vi "check_drift_during_experiment.vi"(8 "error in (no error)":errorcluster, 10 "Processed Image":T1(plugin-control), 11 "max spatial drift since calibration (mm)":dbl) -> (0 "error out":errorcluster, 1 "max spatial drift since experiment start (mm)":sgl, 2 "Image Out":T1, 3 "Warning needed":bool)   [LabVIEW 2019]
uses:
  <vilib>/vision/Image Controls.llb/IMAQ Image.ctl
  ParametersGlobal.vi
  <vilib>/vision/NI_Vision_Development_Module.lvlib
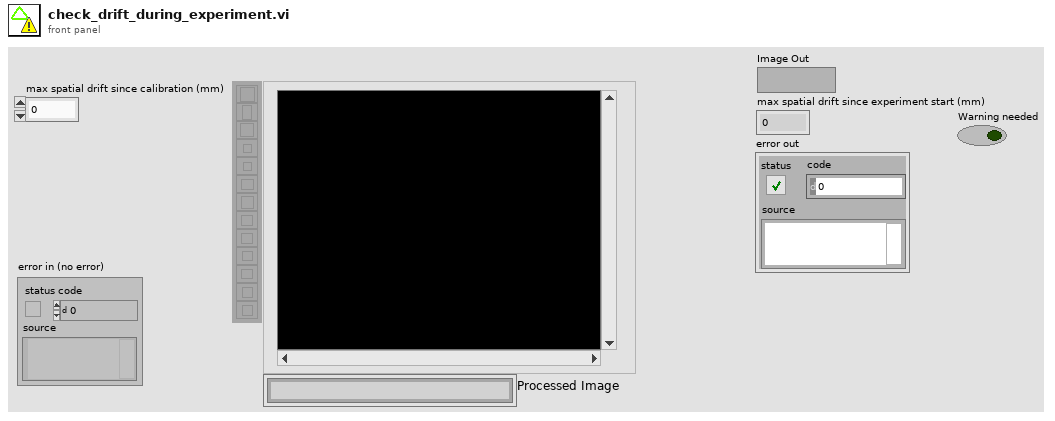
[diagram p1: front panel]
types:
  T1 = typedef "IMAQ Image.ctl" = refnum<image>
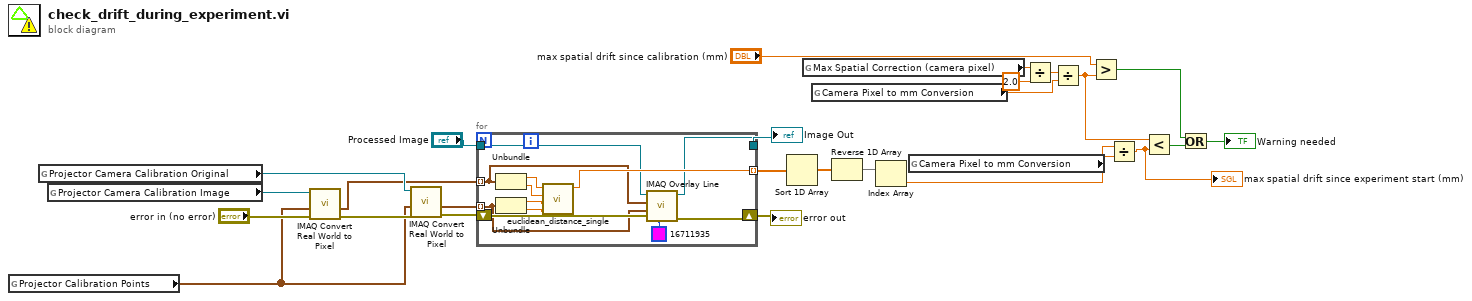
[diagram p0: block diagram]
diagram:
  n1 = global read "ParametersGlobal.vi" "Projector Calibration Points"() -> (w19:cluster{"X":dbl, "Y":dbl}[])
  n2 = global read "ParametersGlobal.vi" "Projector Camera Calibration Original"() -> (w17:T1)
  n3 = global read "ParametersGlobal.vi" "Projector Camera Calibration Image"() -> (w18:T1)
  n4 = call "IMAQ Convert Real World to Pixel"("error in (no error)"="error in (no error)", "Array of Real World Coordinates"=w19, "Calibrated Image"=w18) -> ("error out"=w20:errorcluster, "Array of Pixel Coordinates"=w16:cluster{"X":sgl, "Y":sgl}[])  [unwired: 3 in, 4 out]
  n5 = call "IMAQ Convert Real World to Pixel"("error in (no error)"=w20, "Array of Real World Coordinates"=w19, "Calibrated Image"=w17) -> ("error out"=w11:errorcluster, "Array of Pixel Coordinates"=w15:cluster{"X":sgl, "Y":sgl}[])  [unwired: 3 in, 4 out]
  n6 = for {
    tunnel: w16 -> [w28] mode=indexing
    tunnel: w15 -> [w27] mode=indexing
    tunnel: [w34] -> w12 mode=indexing
    shift-right: [w31] -> w2
    shift-left: w11 -> [w32]
    tunnel: "Processed Image" -> [w30]
    tunnel: [w29] -> w9
    n7 = Unbundle(w28) -> ("X"=w35:sgl, "Y"=w36:sgl)
    n8 = Unbundle(w27) -> ("X"=w37:sgl, "Y"=w38:sgl)
    n9 = call "euclidean_distance_single.vi"("Point 2 Y"=w38, "Point 2 X"=w37, "Point 1 Y"=w36, "Point 1 X"=w35) -> ("Distance"=w34:sgl)  [unwired: 7 in]
    n10 = call "IMAQ Overlay Line"("Color"=u32 16711935, "error in (no error)"=w32, "End Point"=w27, "Start Point"=w28, "Image"=w30) -> ("error out"=w31:errorcluster, "Image Out"=w29:T1)  [unwired: 5 in]
  }
  "Image Out" <- w9
  "error out" <- w2
  n11 = Sort 1D Array(array=w12) -> (sorted array=w14:sgl[])
  n12 = global read "ParametersGlobal.vi" "Max Spatial Correction (camera pixel)"() -> (w22:dbl)
  n13 = global read "ParametersGlobal.vi" "Camera Pixel to mm Conversion"() -> (w26:sgl)
  n14 = Reverse 1D Array(array=w14) -> (reversed array=w13:sgl[])
  n15 = Index Array(array=w13) -> (element=w7:sgl)  [unwired: 1 in]
  n16 = global read "ParametersGlobal.vi" "Camera Pixel to mm Conversion"() -> (w8:sgl)
  n17 = Divide(x=w22, y=2.0) -> (x/y=w25:dbl)
  n18 = Divide(x=w25, y=w26) -> (x/y=w6:dbl)
  n19 = Greater?(x="max spatial drift since calibration (mm)", y=w6) -> (0:w4:bool)
  n20 = Divide(x=w7, y=w8) -> (x/y=w1:sgl)
  "max spatial drift since experiment start (mm)" <- w1
  n21 = Less?(x=w6, y=w1) -> (x < y?=w5:bool)
  n22 = Or(x=w4, y=w5) -> (x .or. y?=→"Warning needed":bool)
